vi "Pointer.Type Cast.vi"() -> ()   [LabVIEW 2016]
uses:
  Source/Classes/Pointer/Memory.Pointer.lvclass/Memory.Pointer.ctl
  Source/Classes/Pointer/Methods/Memory.Pointer.Write.Safe.0D.DBL.vi
  Source/Classes/Pointer/Methods/Memory.Pointer.Read.Safe.0D.U16.vi
  Source/Classes/Pointer/Methods/Memory.Pointer.Write.Safe.0D.U32.vi
  Source/Classes/Pointer/Methods/Memory.Pointer.Read.Safe.0D.U64.vi
  Source/Classes/Pointer/Accessors/Set Address.vi
  Source/Classes/Pointer/Accessors/Set Size.vi
  Source/Classes/Pointer/Accessors/Get Size.vi
  Source/Classes/Pointer/Methods/Memory.Pointer.Copy All.vi
  Source/Classes/Pointer/Methods/Memory.Pointer.Copy All.Safe.vi
  Source/Classes/Pointer/Methods/Memory.Pointer.Write.Unsafe.0D.DBL.vi
  Source/Classes/Pointer/Methods/Memory.Pointer.Parameter Check.Null Pointer.vi
  Source/Classes/Pointer/Methods/Memory.Pointer.Parameter Check.Subset.vi
  Source/Classes/Pointer/Methods/Memory.Pointer.Read.Unsafe.0D.U16.vi
  Source/Classes/Pointer/Accessors/Get Address.vi
  Source/Classes/Pointer/Methods/Memory.Pointer.Write.Unsafe.0D.U32.vi
  Source/Classes/Pointer/Methods/Memory.Pointer.Read.Unsafe.0D.U64.vi
  Source/Classes/Pointer/Methods/Memory.Pointer.Copy.Safe.vi
  Source/Classes/Pointer/Methods/Memory.Pointer.Errors.vi
  Source/Classes/Pointer/Methods/Memory.Pointer.Errors.Null Pointer.vi
  Source/Classes/Pointer/Methods/Memory.Pointer.Errors.Out of Bounds.vi
  Source/Classes/Pointer/Methods/Memory.Pointer.Copy.Unsafe.vi
  Source/Classes/Pointer/Methods/Memory.Pointer.Errors.Create Error.vi
  Source/Submodules/SEH/Source/VIs/Static Error Handling.Source Buffer.Write.String.vi
  Source/Classes/Pointer/Methods/Memory.Pointer.Errors.Write Pointer Size.vi
  Source/Submodules/SEH/Source/VIs/Static Error Handling.Source Buffer.Write.Numeric.Scalar.Base10.vi
  Source/Submodules/SEH/Source/VIs/Static Error Handling.Source Buffer.Write.Numeric.Scalar.Base10 (U64).vi
  Source/Submodules/SEH/Source/VIs/Static Error Handling.Error Cluster Constant.vi
  Source/Submodules/SEH/Source/VIs/Static Error Handling.Error Cluster Constant (256B).vi
  Source/Submodules/SEH/Source/VIs/Static Error Handling.Parameters.Status.Set.vi
  Source/Submodules/SEH/Source/VIs/Static Error Handling.Parameters.Code.Set.vi
  Source/Submodules/SEH/Source/VIs/Static Error Handling.Parameters.VI Source.Set.vi
  Source/Constants/Memory.Constants.vi
  Source/Constants/Memory.Constants.Library Name.vi
  Source/Classes/Pointer/Methods/Memory.Pointer.Errors.Get Info.vi
  Source/Classes/Pointer.Internal/Memory.Pointer.Internal.lvclass
  C:/Users/Ryan/Documents/Git/Sourcetree/LabVIEW-Memory-Manager/Source/Classes/Pointer/Memory.Pointer.lvclass
  Source/Classes/Pointer/Memory.Pointer.lvclass
panel:
  out "unsigned 64bit integer":u64 format="%016x"
  out "*(type *) &x 2":u64 format="%016x"
  out "value out 3":u64 format="%016x"
  out "value":u32 format="%08x"
  out "*(type *) &x":u32 format="%08x"
  out "flatten to string (little-endian)":u16 format="%04x"
  out "lv type cast":u16 format="%04x"
  out "value out":u16 format="%04x"
  in  "byte order":enum16{"big-endian", "little-endian"}(ring)
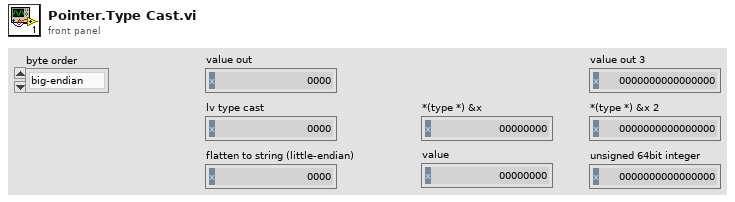
[diagram p1: front panel]
types:
  T1 = enum16{"big-endian, network order", "native, host order", "little-endian"}
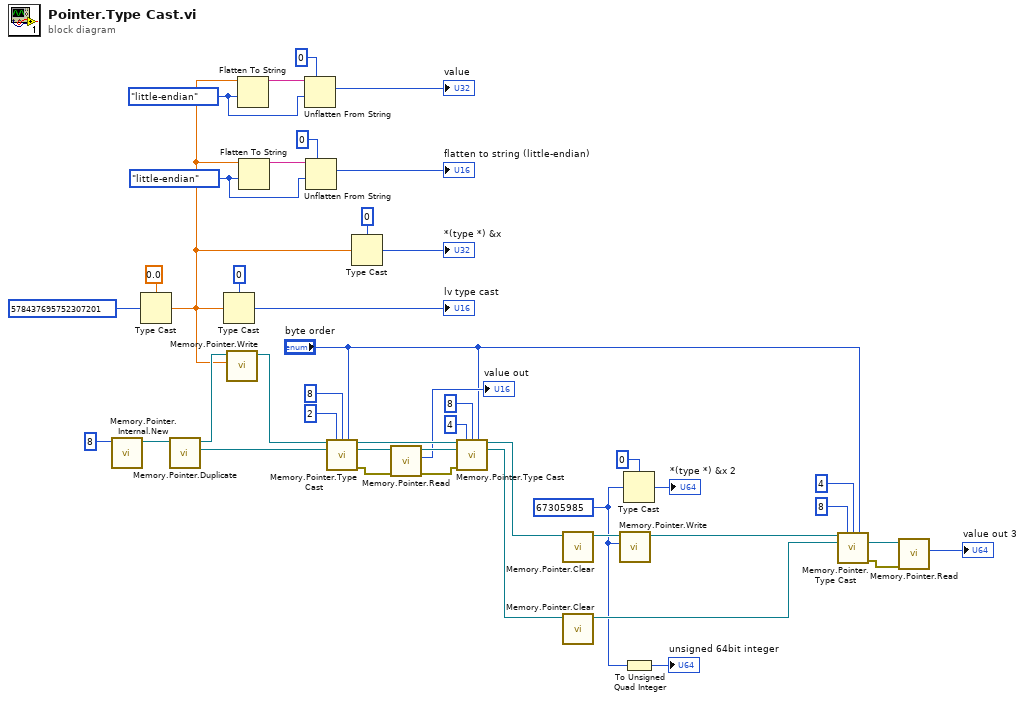
[diagram p0: block diagram]
diagram:
  w1 = u32 67305985
  w20 = T1."little-endian" ("byte order (0:big-endian, network order)")
  w33 = T1."little-endian" ("byte order (0:big-endian, network order)")
  n1 = call "Memory.Pointer.Internal.New.vi"("size"=u64 8) -> ("pointer"=w44:refnum<class "Memory.Pointer.Internal.lvclass">)  [unwired: 9 in, 1 out]
  n2 = Type Cast(type=0.0, x=u64 578437695752307201) -> (*(type *) &x=w18:dbl)
  n3 = call "Memory.Pointer.Duplicate.vi"("pointer in"=w44) -> ("new pointer"=w40:refnum<class "Memory.Pointer.Internal.lvclass">, "pointer out"=w43:refnum<class "Memory.Pointer.Internal.lvclass">)  [unwired: 8 in, 1 out]
  n4 = Type Cast(type=u16 0, x=w18) -> (*(type *) &x=→"lv type cast":u16)
  n5 = call-poly "Memory.Pointer.Write.vi"("value"=w18, "pointer in"=w43) -> ("pointer out"=w39:refnum<class "Memory.Pointer.Internal.lvclass">)  [unwired: 6 in, 3 out]
  n6 = Flatten To String(anything=w18, byte order (0:big-endian, network order)=w20) -> (data string=w19:string)  [unwired: 2 in, 2 out]
  n7 = Flatten To String(anything=w18, byte order (0:big-endian, network order)=w33) -> (data string=w34:string)  [unwired: 2 in, 2 out]
  n8 = Unflatten From String(type=u32 0, binary string=w19, byte order (0:big-endian, network order)=w20) -> (value=→"value":u32)  [unwired: 2 in, 2 out]
  n9 = Unflatten From String(type=u16 0, binary string=w34, byte order (0:big-endian, network order)=w33) -> (value=→"flatten to string (little-endian)":u16)  [unwired: 2 in, 2 out]
  n10 = call "Memory.Pointer.Type Cast.vi"("src pointer in"=w39, "dst width"=u64 2, "src width"=u64 8, "byte order (big-endian)"="byte order", "dst pointer in"=w40) -> ("src pointer out"=w29:refnum<class "Memory.Pointer.Internal.lvclass">, "dst pointer out"=w36:refnum<class "Memory.Pointer.Internal.lvclass">, "error out"=w30:errorcluster)  [unwired: 8 in]
  n11 = Type Cast(type=u32 0, x=w18) -> (*(type *) &x=→"*(type *) &x":u32)
  n12 = call-poly "Memory.Pointer.Read.vi"("error in (no error)"=w30, "pointer in"=w36) -> ("error out"=w16:errorcluster, "value out"=→"value out":u16, "pointer out"=w28:refnum<class "Memory.Pointer.Internal.lvclass">)  [unwired: 6 in, 1 out]
  n13 = call "Memory.Pointer.Type Cast.vi"("src pointer in"=w29, "dst width"=u64 4, "src width"=u64 8, "byte order (big-endian)"="byte order", "dst pointer in"=w28, "error in (no error)"=w16) -> ("src pointer out"=w8:refnum<class "Memory.Pointer.Internal.lvclass">, "dst pointer out"=w6:refnum<class "Memory.Pointer.Internal.lvclass">)  [unwired: 7 in, 1 out]
  n14 = call "Memory.Pointer.Clear.vi"("pointer in"=w8) -> ("pointer out"=w10:refnum<class "Memory.Pointer.Internal.lvclass">)  [unwired: 9 in, 1 out]
  n15 = call "Memory.Pointer.Clear.vi"("pointer in"=w6) -> ("pointer out"=w5:refnum<class "Memory.Pointer.Internal.lvclass">)  [unwired: 9 in, 1 out]
  n16 = call-poly "Memory.Pointer.Write.vi"("value"=w1, "pointer in"=w10) -> ("pointer out"=w7:refnum<class "Memory.Pointer.Internal.lvclass">)  [unwired: 6 in, 3 out]
  n17 = Type Cast(type=u64 0, x=w1) -> (*(type *) &x=→"*(type *) &x 2":u64)
  n18 = To Unsigned Quad Integer(1:w1) -> (0:→"unsigned 64bit integer":u64)
  n19 = call "Memory.Pointer.Type Cast.vi"("src pointer in"=w7, "dst width"=u64 8, "src width"=u64 4, "byte order (big-endian)"="byte order", "dst pointer in"=w5) -> ("dst pointer out"=w13:refnum<class "Memory.Pointer.Internal.lvclass">, "error out"=w11:errorcluster)  [unwired: 8 in, 1 out]
  n20 = call-poly "Memory.Pointer.Read.vi"("error in (no error)"=w11, "pointer in"=w13) -> ("value out"=→"value out 3":u64)  [unwired: 6 in, 3 out]
